vi "Actor Core.vi"(8 "error in":errorcluster, 11 "DLS Laser Actor in":refnum<class "FLS Laser Actor.lvclass">) -> (0 "error out":errorcluster, 3 "Actor out":refnum<class "Actor.lvclass">)   [LabVIEW 2018, in "FLS Laser Actor.lvlib" / "FLS Laser Actor.lvclass"]
doc: "(<B>Filename</B>: Actor Framework.lvlib:Actor.lvclass:Actor Core.vi)\n\nReceives messages to the actor, reacts to them, and initiates any error handling that may shut the actor down.\n\nDescendant classes may override this VI to append parallel tasks for the actor to complete while it handles messages. Overrides use the Call Parent Method node."
uses:
  FLS Laser Actor.lvclass
  C:/Program Files (x86)/National Instruments/LabVIEW 2018/vi.lib/ActorFramework/Actor/Actor.lvclass
  <vilib>/ActorFramework/Actor/Actor.lvclass
  <vilib>/ActorFramework/Actor/Actor.lvclass/Actor.ctl
  <vilib>/ActorFramework/Message Enqueuer/Message Enqueuer.lvclass/Message Enqueuer.ctl
  FLS Laser Actor.lvclass/FLS Laser Actor.ctl
  <vilib>/ActorFramework/Stop Msg/Stop Msg.lvclass/Stop Msg.ctl
  <vilib>/ActorFramework/Message Enqueuer/Init from Existing Queue.vi
  <vilib>/ActorFramework/Message Enqueuer/Enqueue Critical.vi
  <vilib>/ActorFramework/Stop Msg/Stop Msg.lvclass
  C:/Program Files (x86)/National Instruments/LabVIEW 2018/vi.lib/ActorFramework/Message/Message.lvclass
  <vilib>/ActorFramework/Message Priority Queue/Priority Enqueue.vi
  Actor Monitor/Actor/Monitored Actor.lvclass
  <vilib>/ActorFramework/Message Enqueuer/Message Enqueuer.lvclass
  DLS Laser Actor Messages/Measure Range Msg/Measure Range Msg.lvclass
  DLS Laser Actor Messages/Update Fault Indicator Msg/Update Fault Indicator Msg.lvclass
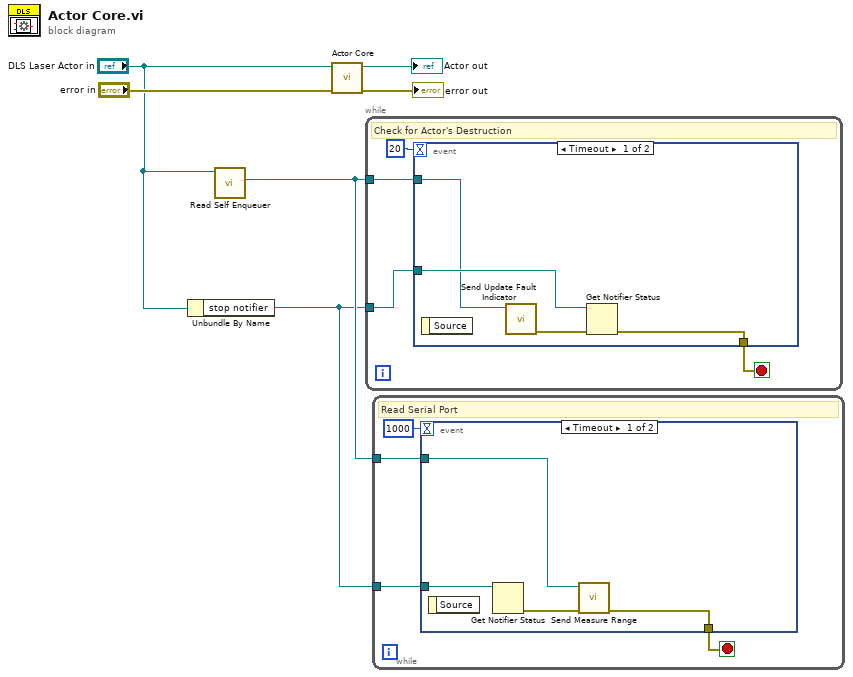
[diagram p0: block diagram]
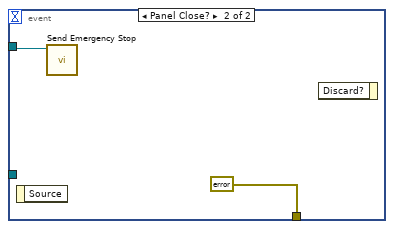
[diagram p2: hidden frame]
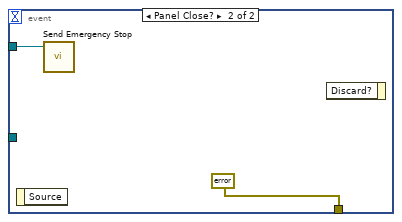
[diagram p3: hidden frame]
diagram:
  n1 = Unbundle By Name("DLS Laser Actor in") -> ("stop notifier"=w1:refnum<notifier>)
  n2 = call <vilib>:"Read Self Enqueuer.vi"("Actor"="DLS Laser Actor in") -> ("Self Enqueuer"=w2:refnum<class "Message Enqueuer.lvclass">)  [unwired: 10 in]
  n3 = call-parent "Actor Core.vi"("error in"="error in", "Actor in"="DLS Laser Actor in") -> ("error out"=→"error out":errorcluster, "Actor out"=→"Actor out":refnum<class "Actor.lvclass">)  [unwired: 8 in]
  n4 = while {
    tunnel: w2 -> [w9]
    tunnel: w1 -> [w8]
    stop <- w7 stop-if-true
    # "Check for Actor's Destruction"
    n5 = event shown="[0] Timeout" {
      selector: _ -> [_ _]
      dyn-events: _ -> [_ _]
      timeout: 20 -> [_ _]
      tunnel: w9 -> [w13 w15]
      tunnel: w8 -> [w14 _]
      tunnel: [w11 errorcluster {"status"=TRUE, "code"=0, "source"=""} ("error out")] -> w7
      event Timeout {
        n6 = event-data() -> ()  [unwired: 1 in, 1 out]
        n7 = call "Send Update Fault Indicator.vi"("Message Enqueuer in"=w13) -> ("error out"=w12:errorcluster)  [unwired: 9 in, 1 out]
        n8 = Get Notifier Status(notifier=w14, error in (no error)=w12) -> (error out=w11:errorcluster)  [unwired: 4 out]
      }
      event Panel Close? {
        n9 = event-data() -> ()  [unwired: 1 in, 1 out]
        n10 = call <vilib>:"Send Emergency Stop.vi"("Message Enqueuer"=w15) -> ()  [unwired: 10 in, 1 out]
        n11 = event-data() -> ()  [unwired: 2 in, 1 out]
      }
    }
  }
  n12 = while {
    tunnel: w2 -> [w19]
    tunnel: w1 -> [w18]
    stop <- w17 stop-if-true
    # "Read Serial Port"
    n13 = event shown="[0] Timeout" {
      selector: _ -> [_ _]
      dyn-events: _ -> [_ _]
      timeout: 1000 -> [_ _]
      tunnel: w19 -> [w23 w25]
      tunnel: w18 -> [w24 _]
      tunnel: [w21 errorcluster {"status"=TRUE, "code"=0, "source"=""} ("error out")] -> w17
      event Timeout {
        n14 = event-data() -> ()  [unwired: 1 in, 1 out]
        n15 = Get Notifier Status(notifier=w24) -> (error out=w22:errorcluster)  [unwired: 1 in, 4 out]
        n16 = call "Send Measure Range.vi"("error in (no error)"=w22, "Message Enqueuer in"=w23) -> ("error out"=w21:errorcluster)  [unwired: 8 in, 1 out]
      }
      event Panel Close? {
        n17 = event-data() -> ()  [unwired: 1 in, 1 out]
        n18 = call <vilib>:"Send Emergency Stop.vi"("Message Enqueuer"=w25) -> ()  [unwired: 10 in, 1 out]
        n19 = event-data() -> ()  [unwired: 2 in, 1 out]
      }
    }
  }
